vi "SEND PUBACK.vi"(8 "error in (no error)":errorcluster, 10 "Message ID":u16=10 format="%x", 11 "connection ID":refnum<k5>) -> (0 "error out":errorcluster, 2 "PubComp Message":u8[](array[numeric]) format="%x", 3 "connection ID out":refnum<k5>)   [LabVIEW 2025, in "DAQIO MQTT.lvlib"]
uses:
  DAQIO MQTT.lvlib
  Controls/MessageType.ctl
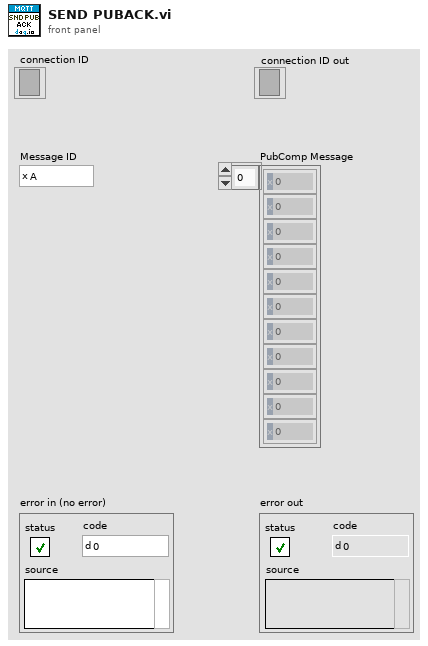
[diagram p1: front panel]
types:
  T1 = typedef "DAQIO MQTT.lvlib/MessageType.ctl" = enum32{"Reserved", "CONNECT", "CONNACK", "PUBLISH", "PUBACK", "PUBREC", "PUBREL", "PUBCOMP", "SUBSCRIBE", "SUBACK", "UNSUBSCRIBE", "UNSUBACK", "PINGREQ", "PINGRESP", "DISCONNECT", "Reserved2"}
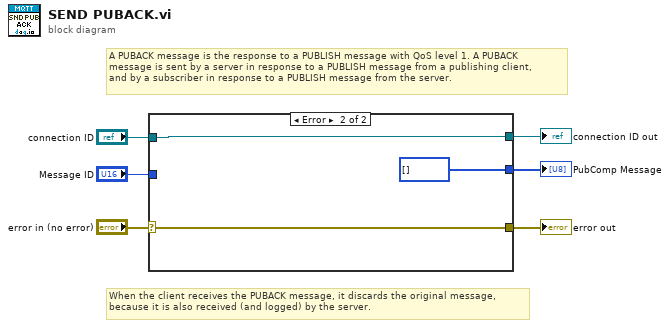
[diagram p0: block diagram]
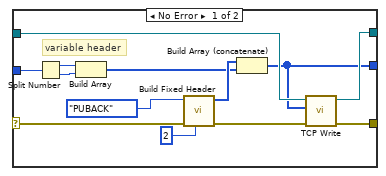
[diagram p2: hidden frame]
diagram:
  # "When the client receives the PUBACK message, it discards the original message,\nbecause it is also received (and logged) by the server."
  # "A PUBACK message is the response to a PUBLISH message with QoS level 1. A PUBACK\nmessage is sent by a server in response to a PUBLISH message from a publishing client,\nand by a subscriber in response to a PUBLISH message from the server."
  n1 = case shown="Error" "error in (no error)" {
    selector: "error in (no error)" -> [w14 w22]
    tunnel: [w12 w22] -> w5
    tunnel: "Message ID" -> [w10 _]
    tunnel: "connection ID" -> [w9 w20]
    tunnel: [w8 w20] -> w2
    tunnel: [w7 u8[] []] -> w1
    frame No Error {
      # "variable header"
      n2 = Split Number(x=w10) -> (hi(x)=w17:u8, lo(x)=w16:u8)
      n3 = Build Array(w17, w16) -> (w13:u8[])
      n4 = call "Build Fixed Header.vi"("Remaining Length"=u32 2, "error in (no error)"=w14, "MessageType"=MessageType."PUBACK") -> ("error out"=w11:errorcluster, "Fixed Header"=w18:u8[])  [unwired: 7 in]
      n5 = Build Array (concatenate)(w18, w13) -> (w7:u8[])
      n6 = call "TCP Write.vi"("error in (no error)"=w11, "data in"=w7, "connection ID"=w9) -> ("error out"=w12:errorcluster, "connection ID out"=w8:refnum<k5>)  [unwired: 6 in, 1 out]
    }
    frame Error {
    }
  }
  "error out" <- w5
  "connection ID out" <- w2
  "PubComp Message" <- w1
